vi "RVHR - Init UI.vi"(6 "Local Data in":T2, 7 "UI Refs":T1, 8 "error in (no error)":errorcluster) -> (0 "error out":errorcluster, 4 "Local Data out":T2)   [LabVIEW 2024]
uses:
  Controls/RVHR - Local Data.ctl
  Controls/Test Cluster.ctl
  Controls/Excluded Information.ctl
  Controls/Language.ctl
  Controls/Device_Type.ctl
  <vilib>/Utility/miscctls.llb/LVRectTypeDef.ctl
  <vilib>/Utility/miscctls.llb/LVBoundsTypeDef.ctl
  Controls/RVHR - UI Refs.ctl
  Buttons/Configure (2).ctl
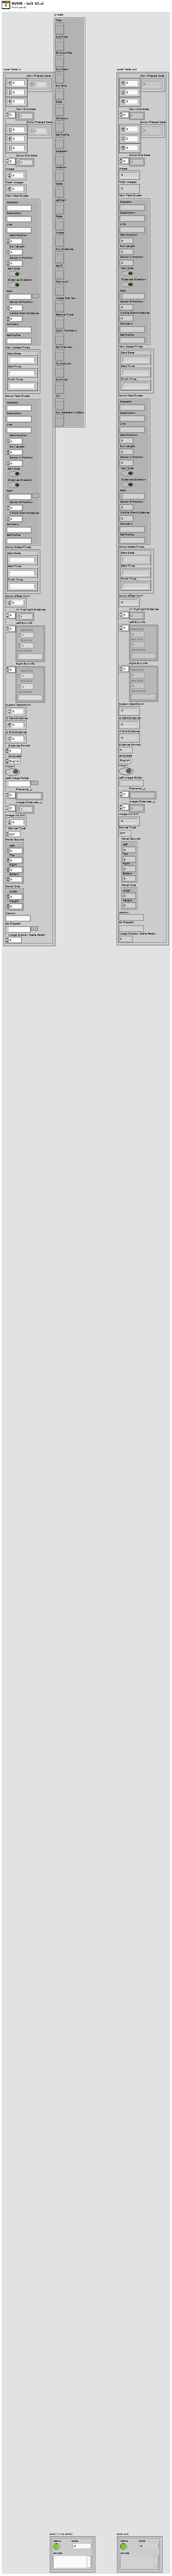
[diagram p1: front panel]
types:
  T1 = typedef "RVHR - UI Refs.ctl" = cluster{"Title":refnum<vi>, "Sub-Title":refnum<vi>, "EN Sub-Title":refnum<vi>, "Run Start":refnum<vi>, "Run End":refnum<vi>, "Date":refnum<vi>, "Company":refnum<vi>, "Ref Profile":refnum<vi>, "Operator":refnum<vi>, "Location":refnum<vi>, "Notes":refnum<vi>, "Left Rail":refnum<vi>, "Page":refnum<vi>, "Image":refnum<vi>, "Run Distance":refnum<vi>, "Next?":refnum<vi>, "Previous?":refnum<vi>, "Image Preview":refnum<vi>, "Feature Type:":refnum<vi>, "Zoom Toolbar L":refnum<vi>, "Rail Preview":refnum<vi>, "ML Analysis":refnum<vi>, "Running?":refnum<vi>, "All?":refnum<vi>, "Run Selection Listbox":refnum<vi>}
  T2 = typedef "RVHR - Local Data.ctl" = cluster{"Main Filtered Data":dbl[][][], "Main Dist Data":dbl[], "Comp Filtered Data":dbl[][][], "Comp Dist Data":dbl[], "Image":u16, "Total Images":u16, "Main Test Cluster":T3, "Main Dates-Times":cluster{"Start Date":string, "Start Time":string, "Finish Time":string}, "Comp Test Cluster":T3, "Comp Dates-Times":cluster{"Start Date":string, "Start Time":string, "Finish Time":string}, "Comp Offset (mm)":i64, "XY Highlight Distance":dbl[], "Left Exc Info":T4[], "Right Exc Info":T4[], "Custom Start-Point":dbl, "UI Start-Distance":dbl, "UI End-Distance":dbl, "Distance Format":u8, "Language":T5, "Vision?":bool, "Left Image Folder":path, "Filename _L":string[], "Image Distances _L":dbl[], "Image Inc (km)":dbl, "Device Type":T6, "Panel Bounds":T7, "Panel Size":T8, "Version":string, "db Filepath":path, "Image Display Scale Factor":dbl}
  T3 = typedef "Test Cluster.ctl" = cluster{"Operator":string, "Description":string, "Line":string, "Start Position":dbl, "Run Length":dbl, "Sensor A Position":dbl, "Rail Side":bool, "Distance Direction":bool, "Path":path, "Sensor B Position":dbl, "Visible Chart Distance":dbl, "Company":string, "Ref Profile":string}
  T4 = typedef "Excluded Information.ctl" = cluster{"Start Dist":dbl, "End Dist":dbl, "Comments":string}
  T5 = typedef "Language.ctl" = enum16{"English", "Chinese", "German"}
  T6 = typedef "Device_Type.ctl" = enum16{"CAT", "Bi-CAT", "YRCA", "RCA", "RV-HR", "TV-HR"}
  T7 = typedef "LVRectTypeDef.ctl" = cluster{"Left":i16, "Top":i16, "Right":i16, "Bottom":i16}
  T8 = typedef "LVBoundsTypeDef.ctl" = cluster{"Width":u32, "Height":u32}
  T9 = cluster{"Start Date":string, "Start Time":string, "Finish Time":string}
  T10 = cluster{"Main Test Cluster":T3, "Main Dates-Times":cluster{"Start Date":string, "Start Time":string, "Finish Time":string}}
  T11 = typedef "Configure (2).ctl" = bool
  T12 = enum8{"Enabled", "Disabled", "Disabled and Grayed Out"}[]
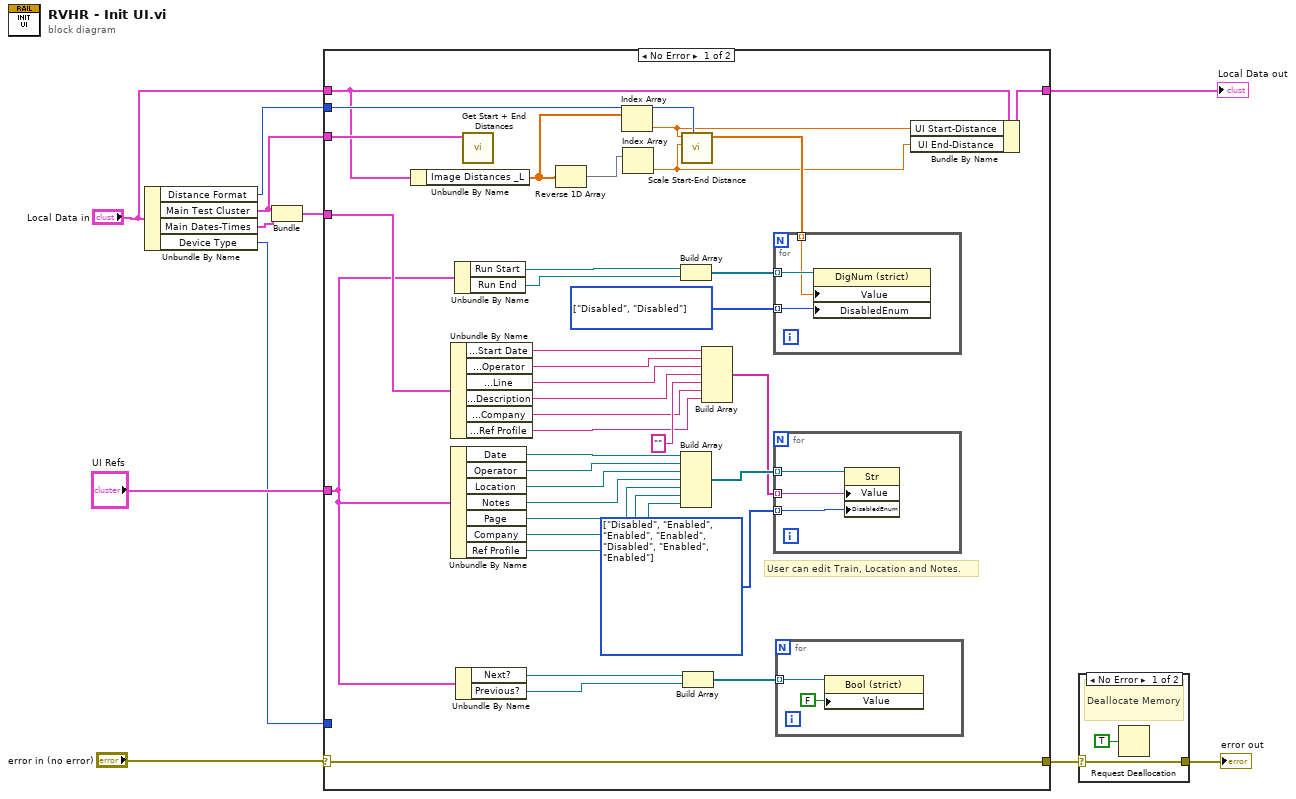
[diagram p0: block diagram]
diagram:
  n1 = Unbundle By Name("Local Data in") -> ("Distance Format"=w6:u8, "Main Test Cluster"=w8:T3, "Main Dates-Times"=w10:T9, "Device Type"=w5:T6)
  n2 = Bundle("Main Test Cluster"=w8, "Main Dates-Times"=w10) -> (w9:T10)  [unwired: 1 in]
  n3 = case shown="No Error" "error in (no error)" {
    selector: "error in (no error)" -> [w47 w57]
    tunnel: [w47 w57] -> w2
    tunnel: "UI Refs" -> [w22 _]
    tunnel: w9 -> [w29 _]
    tunnel: w6 -> [w24 _]
    tunnel: w8 -> [w23 _]
    tunnel: w5 -> [_ _]
    tunnel: "Local Data in" -> [w16 w56]
    tunnel: [w17 w56] -> w3
    frame No Error {
      w30 = T12 [enum."Disabled", enum."Disabled"] items=["Enabled", "Disabled", "Disabled and Grayed Out"]
      w35 = T12 [enum."Disabled", enum."Enabled", enum."Enabled", enum."Enabled", enum."Disabled", enum."Enabled", enum."Enabled"] items=["Enabled", "Disabled", "Disabled and Grayed Out"]
      # "User can edit Train, Location and Notes."
      n4 = Unbundle By Name(w16) -> ("Image Distances _L"=w14:dbl[])
      n5 = Unbundle By Name(w29) -> ("Main Dates-Times.Start Date"=w28:string, "Main Test Cluster.Operator"=w27:string, "Main Test Cluster.Line"=w26:string, "Main Test Cluster.Description"=w25:string, "Main Test Cluster.Company"=w19:string, "Main Test Cluster.Ref Profile"=w18:string)
      n6 = Unbundle By Name(w22) -> ("Date"=w46:refnum<vi>, "Operator"=w37:refnum<vi>, "Location"=w36:refnum<vi>, "Notes"=w45:refnum<vi>, "Page"=w43:refnum<vi>, "Company"=w21:refnum<vi>, "Ref Profile"=w20:refnum<vi>)
      n7 = Unbundle By Name(w22) -> ("Run Start"=w33:refnum<vi>, "Run End"=w34:refnum<vi>)
      n8 = Unbundle By Name(w22) -> ("Next?"=w42:refnum<vi>, "Previous?"=w41:refnum<vi>)
      n9 = call "Get Start + End Distances.vi"("Test Cluster"=w23) -> ()  [unwired: 8 in, 3 out]
      n10 = Reverse 1D Array(array=w14) -> (reversed array=w13:dbl[])
      n11 = Index Array(array=w14) -> (element=w15:dbl)  [unwired: 1 in]
      n12 = Index Array(array=w13) -> (element=w12:dbl)  [unwired: 1 in]
      n13 = Build Array(w33, w34) -> (w32:refnum<vi>[])
      n14 = Build Array(w46, w37, w36, w45, w43, w21, w20) -> (w44:refnum<vi>[])
      n15 = call "Scale Start-End Distance.vi"("Distance Format"=w24, "End Distance"=w12, "Start Distance"=w15) -> ("Start-End Scaled"=w31:dbl[])  [unwired: 8 in]
      n16 = Build Array(w42, w41) -> (w40:refnum<vi>[])
      n17 = Build Array(w28, w27, w26, w25, "" ("element"), w19, w18) -> (w38:string[])
      n18 = for {
        tunnel: w32 -> [w50] mode=indexing
        tunnel: w31 -> [w49] mode=indexing
        tunnel: w30 -> [w48] mode=indexing
        n19 = property class="DigNum (strict)"(reference=w50, "Value"=w49, "DisabledEnum"=w48) -> ()  [unwired: 1 in, 2 out]
      }
      n20 = for {
        tunnel: w44 -> [w53] mode=indexing
        tunnel: w38 -> [w52] mode=indexing
        tunnel: w35 -> [w51] mode=indexing
        n21 = property class="Str"(reference=w53, "Value"=w52, "DisabledEnum"=w51) -> ()  [unwired: 1 in, 2 out]
      }
      n22 = for {
        tunnel: w40 -> [w55] mode=indexing
        n23 = property class="Bool (strict)"(reference=w55, "Value"=T11 FALSE) -> ()  [unwired: 1 in, 2 out]
      }
      n24 = Bundle By Name(cluster=w16, "UI Start-Distance"=w15, "UI End-Distance"=w12) -> (w17:T2)
    }
    frame Error {
    }
  }
  "Local Data out" <- w3
  n25 = case shown="No Error" w2 {
    selector: w2 -> [w58 w60]
    tunnel: [w58 w60] -> w1
    frame No Error {
      # "Deallocate Memory"
      n26 = Request Deallocation(TRUE ("flag")) -> ()
    }
    frame Error {
    }
  }
  "error out" <- w1
